vi "gyro-sweeper-module-V3.vi"(8 "fitter event pair":T4, 9 "async sweeper event pair":T4, 11 "this sweeper event pair":T4) -> ()   [LabVIEW 2018]
uses:
  filename-pattern.ctl
  show-win- control.ctl
  cursor winow.ctl
  server talk-to-back pair.ctl
  server talkback message type.ctl
  server talkto message type.ctl
  cursor window action.ctl
  pll internal user event action.ctl
  publisher action.ctl
  file -- read-write control.ctl
  KM_file -- read-write control.ctl
  filename-action.ctl
  <vilib>/Analysis/baseanly.llb/A x B.vi
  <vilib>/Analysis/baseanly.llb/Complex A x B.vi
  Q -- check range -- i -- real.vi
  line -- complex.vi
  Q -- check range -- i -- integer.vi
  Q - not nan -- real.vi
  Q - not nan -- integer.vi
  <vilib>/Analysis/Matrix/Numeric/Conversions/Array To Matrix.vi
  <vilib>/Analysis/Matrix/Numeric/Conversions/Array To Matrix - RA2.vi
  <vilib>/Analysis/baseanly.llb/Inverse Matrix.vi
  <vilib>/Analysis/baseanly.llb/Real Inverse Matrix.vi
panel:
  in  "view/hide fitter":bool
  in  "view/hide sweeper":bool=TRUE
  in  "sweeper panel":T1(tab)
  in  "sweep ON":bool
  in  "win":T2={"cen (Hz)"=32744.4, "win (Hz)"=134.34356253945762, "left (Hz)"=32677.228218730274, "right (Hz)"=32811.57178126973}
  out "Plot: circle sweep window":cluster{"Freq out (Hz)":dbl[], dbl[]}[](graph)
  in  "start/stop sweep: r":bool
  in  "subtract bgnd!":bool
  in  "fit!":bool=TRUE
  in  "cursor window":T3={"left"=32677.228218730274, "right "=32811.57178126973, "center"=32744.4, "window"=134.34356253945762, "cursors"=[0, 1, 2], "relative"=0, "absolute"=0, "fixed vertical offset"=0.0, "vertical offset"=0.0, "skew"=0.0, "default window frac"=0.1, "kind"=enum."symmetric", "skew.left"=0.5, "skew.right"=0.5, "Plot ref"=refnum, "wing order"=enum."forw"}
  in  "save data":enum32{"save/read"}(tab)
  in  "freqsweep name template":T5={"prefix"="RuCl3-rod", "group"="f"}
  in  "Save folder":path=path "/Users/Shared/Data"
  in  "freq sweep file name":string="f020_RuCl3-rod_042518.dat"
  in  "read from disk :l":bool
  in  "read file":path=path "/Users/arkady/Desktop/local_data/TaAs-quirk-Jan2018-losalamos/9w/f006_rucl3_012518.dat"
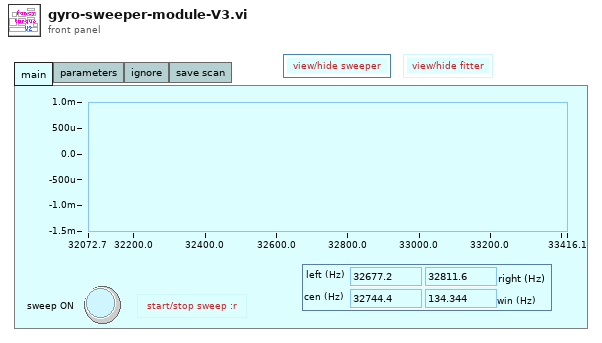
[diagram p1: front panel]
types:
  T1 = enum32{"main", "parameters", "ignore", "save scan"}
  T2 = typedef "show-win- control.ctl" = cluster{"cen (Hz)":dbl, "win (Hz)":dbl, "left (Hz)":dbl, "right (Hz)":dbl}
  T3 = typedef "cursor winow.ctl" = cluster{"left":dbl, "right ":dbl, "center":dbl, "window":dbl, "cursors":i32[], "relative":i32, "absolute":i32, "fixed vertical offset":dbl, "vertical offset":dbl, "skew":dbl, "default window frac":dbl, "kind":enum16{"symmetric", "skewed", "fancy"}, "skew.left":dbl, "skew.right":dbl, "Plot ref":refnum<vi>, "wing order":enum16{"forw", "back"}}
  T4 = typedef "server talk-to-back pair.ctl" = cluster{"talkback event":refnum<user-event>, "talkto event":refnum<user-event>}
  T5 = typedef "filename-pattern.ctl" = cluster{"prefix":string, "group":string}
  T6 = typedef "pll internal user event action.ctl" = enum16{"gear pll async", "start pll async", "stop pll async", "toggle pll async", "gear sweeper", "start sweeper", "stop sweeper", "toggle sweeper", "accept frequency", "reset lorentzian", "accept lorentzian", "update cursors", "pause pll", "unpause pll", "void", "exit", "gear server sweeper", "gear sweeper async", "gear fitter", "gear sourcer"}
  T7 = typedef "cursor window action.ctl" = enum16{"balance", "h. offset change", "cursor moves", "change center", "change window", "init", "check", "reset", "set y to middle", "idle", "-write all Y", "-write left.X", "-write center.X", "-write right.X", "-write all X", "-change center", "-change window", "-change skew", "-read cursor 2", "-read cursor 1", "-read cursor 0", "-read all cursors", "-reset", "-read plot scale", "-set y to middle", "-Q: center.Y is visible", "-Q: window is visible", "-parse center.Y", "-right left from center", "-left move", "-right move", "-set center.Y", "-empty", "-set cursors to default", "-check", "-write center.Y", "-copy cursor 1", "-copy cursor 0", "-copy cursor 2", "move right", "move left", "shrink", "broaden", "skew up", "skew down", "-write plot scale", "zoom X", "change cen&win", "zoom to all data", "color--red", "color--green", "color--yellow", "read", "zoom out", "zoom in", "slide right", "slide left", "set range aspect ratio to 1"}
  T8 = enum16{"stop", "start", "update pars", "update request", "new", "launch", "exit", "get", "reset", "pause", "unpause"}
  T9 = typedef "publisher action.ctl" = enum16{"set", "get", "init", "check"}
  T10 = typedef "file -- read-write control.ctl" = enum16{"read", "write all", "append one line"}
  T11 = typedef "filename-action.ctl" = enum16{"rewrite", "parse", "force pattern", "uniquenum"}
  T12 = typedef "KM_file -- read-write control.ctl" = enum16{"read", "write all", "append one line"}
  T13 = typedef "server talkto message type.ctl" = cluster{"message":enum16{"stop", "start", "update pars", "update request", "new", "launch", "exit", "get", "reset", "pause", "unpause"}}
  T14 = typedef "eventvkey.ctl" = enum16{"ASCII", "Enter", "Return", "Shift", "Ctrl", "Alt", "Cmd", "Opt", "Caps", "NumLock", "Clear", "Break", "Up", "Down", "Left", "Right", "Insert", "Delete", "Home", "End", "PageUp", "PageDown", "Escape", "Help", "Pause", "ScrollLock", "F1", "F2", "F3", "F4", "F5", "F6", "F7", "F8", "F9", "F10", "F11", "F12", "F13", "F14", "F15", "F16", "F17", "F18", "F19", "F20", "F21", "F22", "F23", "F24", "Play", "VolumeUp", "VolumeDown", "Mute", "Two Byte Char"}
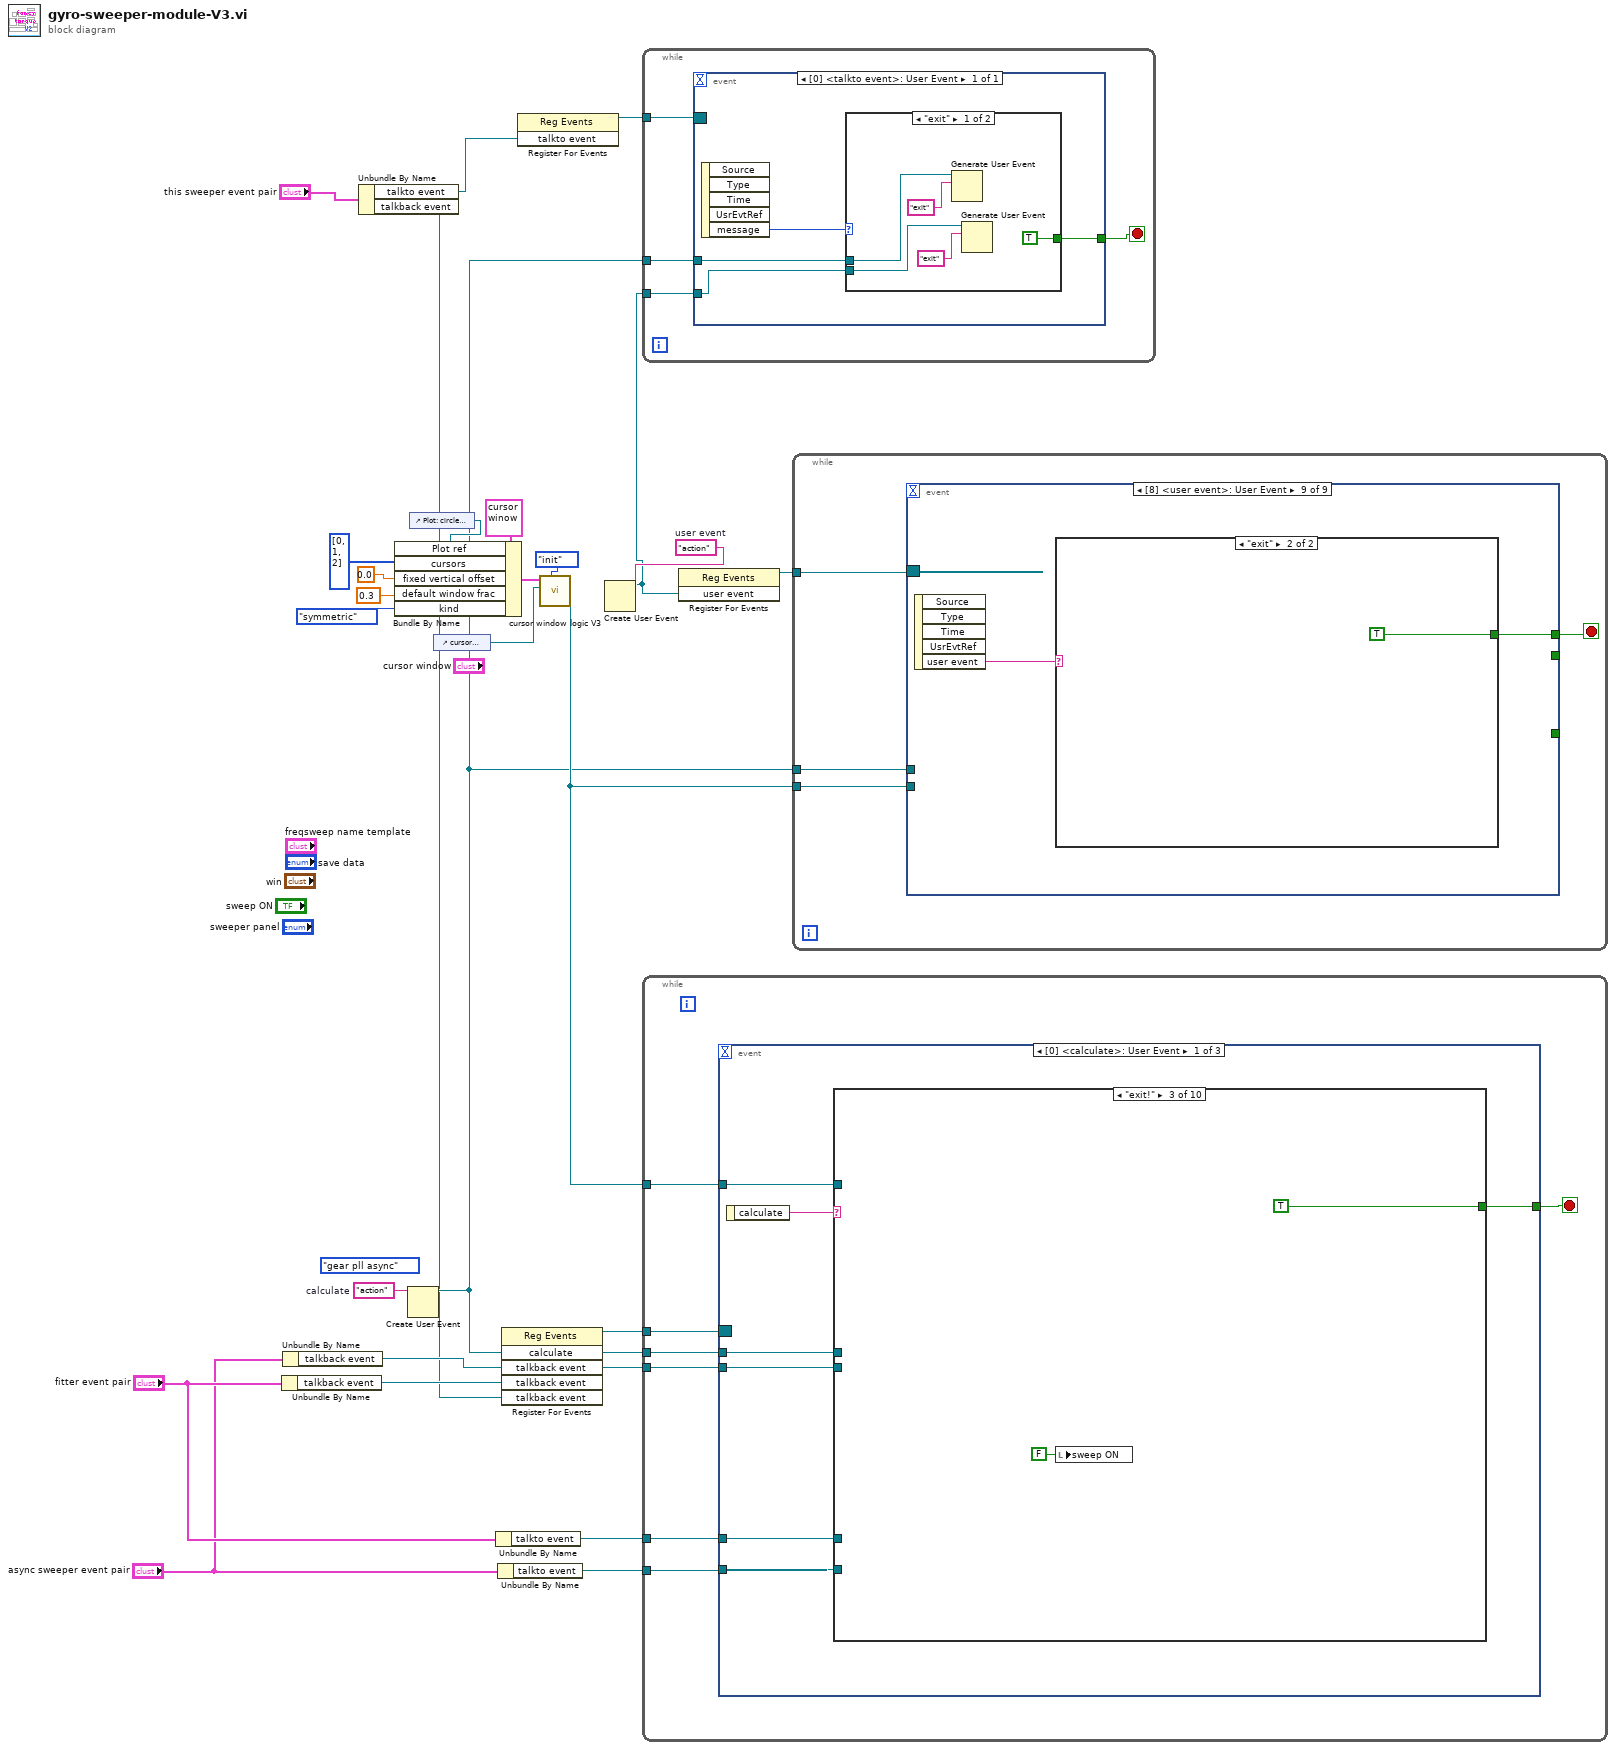
[diagram p0: block diagram]
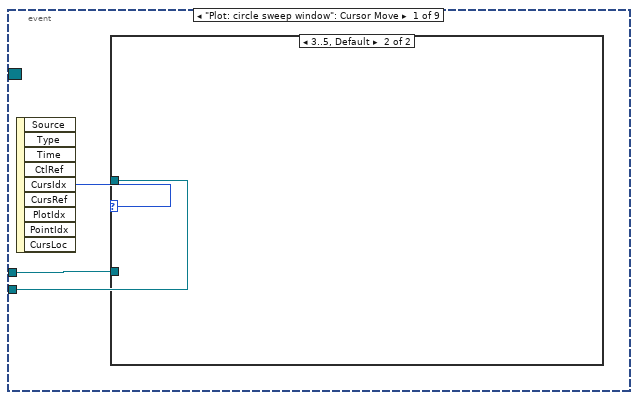
[diagram p3: hidden frame]
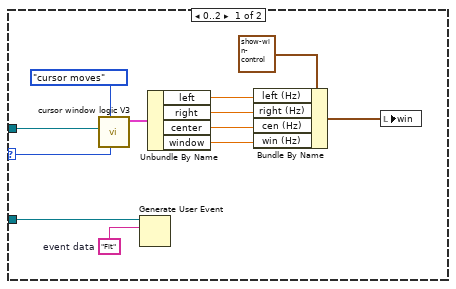
[diagram p4: hidden frame]
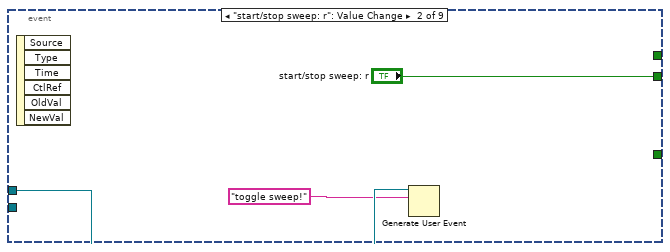
[diagram p5: hidden frame]
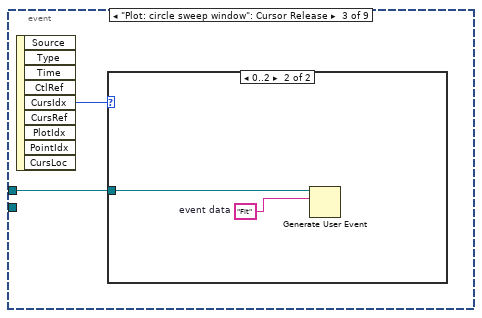
[diagram p6: hidden frame]
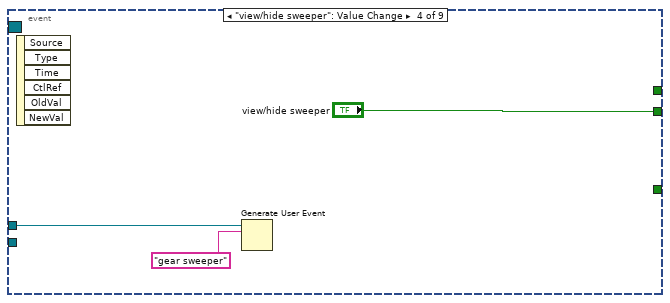
[diagram p8: hidden frame]
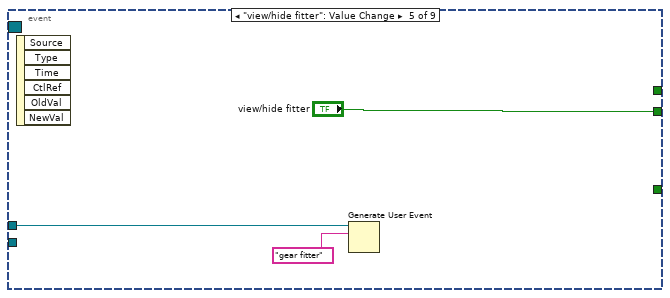
[diagram p9: hidden frame]
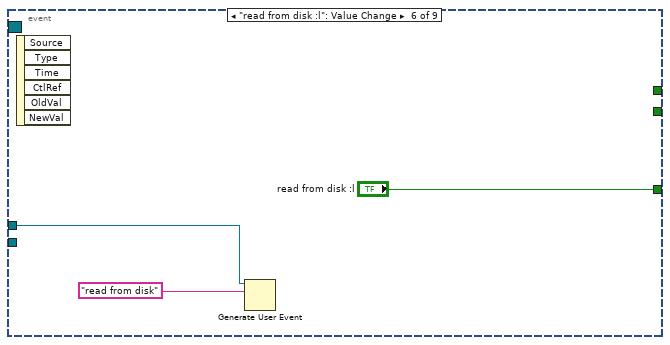
[diagram p10: hidden frame]
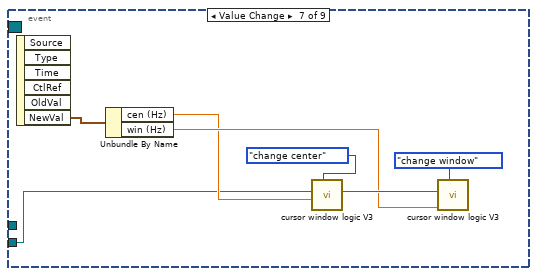
[diagram p11: hidden frame]
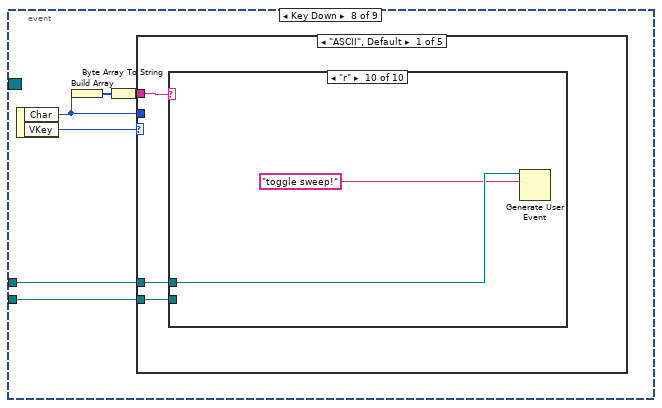
[diagram p12: hidden frame]
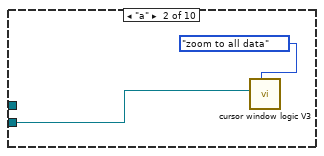
[diagram p14: hidden frame]
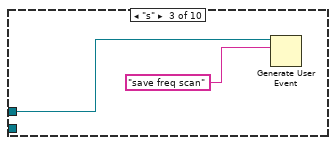
[diagram p15: hidden frame]
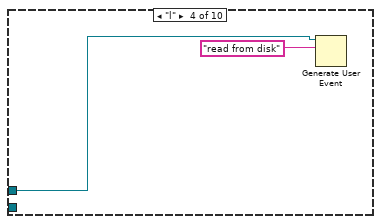
[diagram p16: hidden frame]
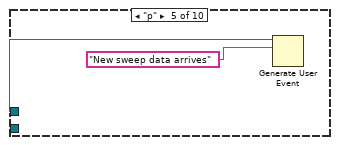
[diagram p17: hidden frame]
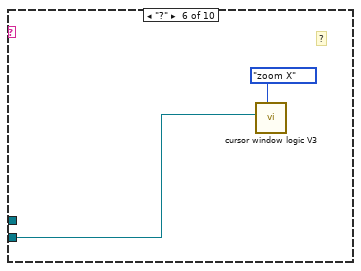
[diagram p18: hidden frame]
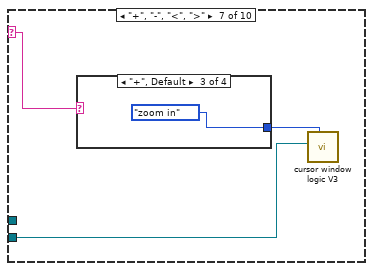
[diagram p19: hidden frame]
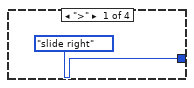
[diagram p20: hidden frame]
diagram:
  (unwired) pll_internal_user_event_action."gear pll async" ("pll event action")
  w23 = "action"  # user event
  w25 = "action"  # calculate
  n1 = Unbundle By Name("fitter event pair") -> ("talkback event"=w9:refnum<user-event>)
  n2 = Unbundle By Name("async sweeper event pair") -> ("talkback event"=w7:refnum<user-event>)
  n3 = Unbundle By Name("this sweeper event pair") -> ("talkto event"=w4:refnum<user-event>, "talkback event"=w1:refnum<user-event>)
  n4 = Create User Event(user event datatype=w25) -> (user event=w2:refnum<user-event>)  [unwired: 1 in, 1 out]
  n5 = control-ref of="Plot: circle sweep window"() -> (w14:refnum<vi>)
  n6 = Bundle By Name(cluster=T3 {"left"=0.0, "right "=0.0, "center"=0.0, "window"=0.0, "cursors"=[], "relative"=0, "absolute"=0, "fixed vertical offset"=0.0, "vertical offset"=0.0, "skew"=0.0, "default window frac"=0.0, "kind"=enum."symmetric", "skew.left"=0.0, "skew.right"=0.0, "Plot ref"=refnum, "wing order"=enum."forw"} ("cursor bracket: All, data window"), "Plot ref"=w14, "cursors"=i32[] [0, 1, 2], "fixed vertical offset"=0.0, "default window frac"=0.3 ("fixed vertical offset"), "kind"=enum16{"symmetric", "skewed", "fancy"}."symmetric") -> (w18:T3)
  n7 = control-ref of="cursor window"() -> (w13:refnum<vi>)
  n8 = Unbundle By Name("fitter event pair") -> ("talkto event"=w11:refnum<user-event>)
  n9 = Unbundle By Name("async sweeper event pair") -> ("talkto event"=w12:refnum<user-event>)
  n10 = register-events(w2, w7, w9, w1) -> (reference out=w26:refnum<event-registration>)  [unwired: 2 in, 1 out]
  n11 = register-events(w4) -> (reference out=w6:refnum<event-registration>)  [unwired: 2 in, 1 out]
  n12 = call "cursor window logic V3.vi"("cursor window action"=cursor_window_action."init", "cursor window in"=w13, "cursor window init"=w18) -> ("cursor window out"=w16:refnum<vi>)  [unwired: 7 in, 1 out]
  n13 = Create User Event(user event datatype=w23) -> (user event=w3:refnum<user-event>)  [unwired: 1 in, 1 out]
  n14 = while {
    tunnel: w6 -> [w30]
    tunnel: w2 -> [w28]
    tunnel: w3 -> [w27]
    stop <- w29 stop-if-true
    n15 = event shown="[0] <talkto event>: User Event" {
      selector: w30 -> [_]
      dyn-events: _ -> [_]
      timeout: _ -> [_]
      tunnel: [w33] -> w29
      tunnel: w28 -> [w32]
      tunnel: w27 -> [w31]
      event User Event {
        n16 = event-data() -> ("message"=w34:T8)  [unwired: 1 in, 4 out]
        n17 = case shown="\"exit\"" w34 {
          tunnel: [TRUE _] -> w33
          tunnel: w32 -> [w38 _]
          tunnel: w31 -> [w35 _]
          frame "exit" {
            n18 = Generate User Event(user event=w38, event data cluster="exit" ("event data")) -> ()  [unwired: 2 in, 2 out]
            n19 = Generate User Event(user event=w35, event data cluster="exit" ("event data")) -> ()  [unwired: 2 in, 2 out]
          }
          frame "start", Default {
          }
        }
      }
    }
  }
  n20 = while {
    tunnel: w26 -> [w46]
    tunnel: w2 -> [w45]
    tunnel: w16 -> [w44]
    tunnel: w12 -> [w43]
    tunnel: w7 -> [w42]
    tunnel: w11 -> [w41]
    stop <- w40 stop-if-true
    n21 = event shown="[0] <calculate>: User Event" {
      selector: w46 -> [_ _ _]
      dyn-events: _ -> [_ _ _]
      timeout: _ -> [_ _ _]
      tunnel: w45 -> [w52 w145 _]
      tunnel: w44 -> [w51 _ _]
      tunnel: w43 -> [w50 _ _]
      tunnel: w42 -> [w49 _ _]
      tunnel: w41 -> [w48 _ _]
      tunnel: [w47 _ _] -> w40
      event User Event {
        n22 = event-data() -> ("calculate"=w53:string)  [unwired: 1 in]
        n23 = case shown="\"exit!\"" w53 {
          tunnel: w52 -> [w62 w85 _ w90 _ _ _ _ _ _]
          tunnel: w51 -> [_ _ _ _ _ w122 _ _ _ _]
          tunnel: w50 -> [_ _ _ _ _ _ w135 w140 w144 _]
          tunnel: w49 -> [_ _ _ _ _ _ _ _ _ _]
          tunnel: w48 -> [_ _ _ _ _ w120 _ _ _ _]
          tunnel: [_ _ TRUE _ _ _ _ _ _ _] -> w47
          frame "New sweep data arrives" {
            n24 = call "MFLI -- publish -- freq scan.vi"("publisher action"=publisher_action."get") -> ("Voltage out (V)"=w59:cdb[], "Freq out (Hz)"=w61:dbl[])  [unwired: 9 in]
            n25 = Generate User Event(user event=w62, event data cluster="Fit" ("event data")) -> ()  [unwired: 2 in, 2 out]
            n26 = case shown="False" "subtract bgnd!" {
              tunnel: w61 -> [w74 w82]
              tunnel: [w68 w82] -> w60
              tunnel: w59 -> [w70 w81]
              tunnel: [w75 w81] -> w58
              frame True {
                w67 = 10 ("length")
                n27 = Delete From Array(array=w74, length=w67, index=0) -> (array with subset deleted=w73:dbl[])  [unwired: 1 out]
                n28 = Delete From Array(array=w70, length=w67, index=0) -> (array with subset deleted=w69:cdb[])  [unwired: 1 out]
                n29 = call "linear interp iiii- complex - z-omega.vi"("z"=w69, "omega"=w73) -> ("z out"=w76:cdb[], "omega out"=w68:dbl[], "intercept"=w78:cdb, "slope"=w79:cdb)  [unwired: 5 in, 5 out]
                n30 = Multiply(x=w68, y=w79) -> (x*y=w80:cdb[])
                n31 = Add(x=w80, y=w78) -> (x+y=w77:cdb[])
                n32 = Subtract(x=w76, y=w77) -> (x-y=w75:cdb[])
              }
              frame False {
              }
            }
            n33 = Complex To Re/Im(x + iy=w58) -> (x=w65:dbl[], y=w64:dbl[])
            n34 = Bundle("Freq out (Hz)"=w60, w65) -> (w66:cluster{"Freq out (Hz)":dbl[], dbl[]})  [unwired: 1 in]
            n35 = Bundle("Freq out (Hz)"=w60, w64) -> (w63:cluster{"Freq out (Hz)":dbl[], dbl[]})  [unwired: 1 in]
            n36 = Build Array(w66, w63) -> (→"Plot: circle sweep window":cluster{"Freq out (Hz)":dbl[], dbl[]}[])
          }
          frame "toggle sweep!" {
            n37 = local read "sweep ON"() -> (w84:bool)
            n38 = case shown="False" w84 {
              tunnel: ["start sweep!" ("event data") "stop sweep!" ("event data")] -> w83
              frame False {
              }
              frame True {
              }
            }
            n39 = Generate User Event(user event=w85, event data cluster=w83) -> ()  [unwired: 2 in, 2 out]
          }
          frame "exit!" {
            n40 = local write "sweep ON"(FALSE ("sweep ON")) -> ()
          }
          frame "read from disk" {
            n41 = call "file - read-write - list of lines.vi"("read/write control"=file_--_read-write_control."read", "file path"="read file") -> ("list of lines OUT"=w94:string[])  [unwired: 8 in, 1 out]
            n42 = for {
              tunnel: w94 -> [w104] mode=indexing
              tunnel: [w99] -> w95 mode=indexing
              tunnel: [w98] -> w96 mode=indexing
              w100 = 0.0
              n43 = Scan From String(format string="%f%f%f", input string=w104, default 1=w100, default 2=w100, default 3=w100) -> (output 1=w98:dbl, output 2=w102:dbl, output 3=w101:dbl)  [unwired: 2 in, 3 out]
              n44 = Re/Im To Complex(1:w101, 2:w102) -> (0:w99:cdb)
            }
            n45 = flat-sequence {
              tunnel: w90 -> [w108]
              tunnel: [w108] -> w97
              tunnel: w95 -> [w106]
              tunnel: w96 -> [w105]
              tunnel: w97 -> [w110]
              tunnel: "New sweep data arrives" ("event data") -> [w109]
              frame #0 {
                n46 = call "MFLI -- publish -- freq scan.vi"("publisher action"=publisher_action."set", "Voltage IN (V)"=w106, "Freq IN (Hz)"=w105) -> ()  [unwired: 7 in, 2 out]
              }
              frame #1 {
                n47 = Generate User Event(user event=w110, event data cluster=w109) -> ()  [unwired: 2 in, 2 out]
              }
            }
          }
          frame "save freq scan" {
            n48 = local read "freqsweep name template"() -> (w116:T5)
            n49 = call "MFLI -- publish -- freq scan.vi"("publisher action"=publisher_action."get") -> ("Voltage out (V)"=w112:cdb[], "Freq out (Hz)"=w113:dbl[])  [unwired: 9 in]
            n50 = call "filename-manage.vi"("filename pattern"=w116, "filename-action"=filename-action."uniquenum", "folder"="Save folder", "file name"="freq sweep file name") -> ("filename OUT"=w115:string)  [unwired: 7 in]
            n51 = call "KM_appendline -- freq sweep.vi"("freq"=w113, "Vout(V)"=w112, "Save frequency scan"="Save folder", "read/write control"=KM_file_--_read-write_control."append one line", "name or relative path"=w115) -> ()  [unwired: 15 in]
            n52 = local write "freq sweep file name"(w115) -> ()
          }
          frame "Fit" {
            n53 = case shown="True" "fit!" {
              tunnel: w122 -> [_ w124]
              tunnel: w120 -> [_ w123]
              frame False {
              }
              frame True {
                n54 = flat-sequence {
                  tunnel: w124 -> [w127]
                  tunnel: w123 -> [w129]
                  frame #0 {
                    n55 = call "cursor window logic V3.vi"("cursor window action"=cursor_window_action."read", "cursor window in"=w127) -> ("cursor window out"=w126:T3)  [unwired: 8 in, 1 out]
                    n56 = call "publish -- fitter window.vi"("publisher action"=publisher_action."set", "win IN"=w126) -> ()  [unwired: 9 in, 1 out]
                  }
                  frame #1 {
                    n57 = Generate User Event(user event=w129, event data cluster=T13 {"message"=enum."new"} ("event data")) -> ()  [unwired: 2 in, 2 out]
                  }
                }
              }
            }
          }
          frame "start sweep!" {
            n58 = local read "win"() -> (w132:T2)
            n59 = call "publish -- sweeper window.vi"("publisher action"=publisher_action."set", "win IN"=w132) -> ()  [unwired: 9 in, 1 out]
            n60 = local write "sweep ON"(TRUE ("sweep ON")) -> ()
            n61 = Generate User Event(user event=w135, event data cluster=T13 {"message"=enum."update request"} ("event data")) -> (user event out=w134:refnum<user-event>)  [unwired: 2 in, 1 out]
            n62 = Generate User Event(user event=w134, event data cluster=T13 {"message"=enum."start"} ("event data")) -> ()  [unwired: 2 in, 2 out]
          }
          frame "stop sweep!" {
            n63 = Generate User Event(user event=w140, event data cluster=T13 {"message"=enum."stop"} ("event data")) -> ()  [unwired: 2 in, 2 out]
            n64 = local write "sweep ON"(FALSE ("sweep ON")) -> ()
          }
          frame "update win" {
            n65 = local read "win"() -> (w141:T2)
            n66 = call "publish -- sweeper window.vi"("publisher action"=publisher_action."set", "win IN"=w141) -> ()  [unwired: 9 in, 1 out]
            n67 = Generate User Event(user event=w144, event data cluster=T13 {"message"=enum."update request"} ("event data")) -> ()  [unwired: 2 in, 2 out]
          }
          frame "Void", Default {
          }
        }
      }
      event User Event {
        n68 = event-data() -> ("message"=w146:enum16{"new", "void"})  [unwired: 1 in, 4 out]
        n69 = case shown="\"new\", Default" w146 {
          tunnel: w145 -> [w147]
          frame "new", Default {
            n70 = Generate User Event(user event=w147, event data cluster="New sweep data arrives" ("event data")) -> ()  [unwired: 2 in, 2 out]
          }
        }
      }
      event User Event {
        n71 = event-data() -> ()  [unwired: 1 in, 1 out]
      }
    }
  }
  n72 = register-events(w3) -> (reference out=w24:refnum<event-registration>)  [unwired: 2 in, 1 out]
  n73 = while {
    tunnel: w24 -> [w152]
    tunnel: w2 -> [w151]
    tunnel: w16 -> [w150]
    stop <- w149 stop-if-true
    n74 = event shown="[8] <user event>: User Event" {
      selector: w152 -> [_ _ _ _ _ _ _ _ _]
      dyn-events: _ -> [_ _ _ _ _ _ _ _ _]
      timeout: _ -> [_ _ _ _ _ _ _ _ _]
      tunnel: w151 -> [w153 w169 w172 w176 w178 w183 _ w195 _]
      tunnel: w150 -> [w155 _ _ _ _ _ w184 w191 _]
      tunnel: [_ "start/stop sweep: r" _ "view/hide sweeper" "view/hide fitter" _ _ _ _] -> _
      tunnel: [_ _ _ _ _ "read from disk :l" _ _ _] -> _
      tunnel: [_ _ _ _ _ _ _ _ w239] -> w149
      event "Plot: circle sweep window": Cursor Move {
        n75 = event-data() -> ("CursIdx"=w154:i32)  [unwired: 1 in, 8 out]
        n76 = case shown="3..5, Default" w154 {
          selector: w154 -> [w165 _]
          tunnel: w155 -> [w167 _]
          tunnel: w153 -> [w163 _]
          frame 0..2 {
            w162 = "Fit"  # event data
            n77 = call "cursor window logic V3.vi"("CursIdx"=w165, "cursor window action"=cursor_window_action."cursor moves", "cursor window in"=w167) -> ("cursor window out"=w164:T3)  [unwired: 7 in, 1 out]
            n78 = Generate User Event(user event=w163, event data cluster=w162) -> ()  [unwired: 2 in, 2 out]
            n79 = Unbundle By Name(w164) -> ("left"=w159:dbl, "right"=w158:dbl, "center"=w157:dbl, "window"=w156:dbl)
            n80 = Bundle By Name(cluster=T2 {"cen (Hz)"=-0.35260838541595674, "win (Hz)"=17.234446484426172, "left (Hz)"=-8.969831627629043, "right (Hz)"=8.26461485679713} ("win"), "left (Hz)"=w159, "right (Hz)"=w158, "cen (Hz)"=w157, "win (Hz)"=w156) -> (w160:T2)
            n81 = local write "win"(w160) -> ()
          }
          frame 3..5, Default {
          }
        }
      }
      event "start/stop sweep: r": Value Change {
        n82 = event-data() -> ()  [unwired: 1 in, 6 out]
        n83 = Generate User Event(user event=w169, event data cluster="toggle sweep!" ("event data")) -> ()  [unwired: 2 in, 2 out]
      }
      event "Plot: circle sweep window": Cursor Release {
        n84 = event-data() -> ("CursIdx"=w171:i32)  [unwired: 1 in, 8 out]
        n85 = case shown="0..2" w171 {
          tunnel: w172 -> [_ w173]
          frame 3, Default {
          }
          frame 0..2 {
            w174 = "Fit"  # event data
            n86 = Generate User Event(user event=w173, event data cluster=w174) -> ()  [unwired: 2 in, 2 out]
          }
        }
      }
      event "view/hide sweeper": Value Change {
        n87 = event-data() -> ()  [unwired: 1 in, 6 out]
        n88 = Generate User Event(user event=w176, event data cluster="gear sweeper" ("event data")) -> ()  [unwired: 2 in, 2 out]
      }
      event "view/hide fitter": Value Change {
        n89 = event-data() -> ()  [unwired: 1 in, 6 out]
        n90 = Generate User Event(user event=w178, event data cluster="gear fitter" ("event data")) -> ()  [unwired: 2 in, 2 out]
      }
      event "read from disk :l": Value Change {
        n91 = event-data() -> ()  [unwired: 1 in, 6 out]
        n92 = Generate User Event(user event=w183, event data cluster="read from disk" ("event data")) -> ()  [unwired: 2 in, 2 out]
      }
      event Value Change {
        n93 = event-data() -> ("NewVal"=w187:T2)  [unwired: 1 in, 5 out]
        n94 = Unbundle By Name(w187) -> ("cen (Hz)"=w185:dbl, "win (Hz)"=w186:dbl)
        n95 = call "cursor window logic V3.vi"("cursor window action"=cursor_window_action."change center", "center"=w185, "cursor window in"=w184) -> ("cursor window out"=w188:refnum<vi>)  [unwired: 7 in, 1 out]
        n96 = call "cursor window logic V3.vi"("cursor window action"=cursor_window_action."change window", "window"=w186, "cursor window in"=w188) -> ()  [unwired: 7 in, 2 out]
      }
      event Key Down {
        n97 = event-data() -> ("Char"=w193:i16, "VKey"=w196:T14)  [unwired: 1 in]
        n98 = Build Array(w193) -> (w194:i16[])
        n99 = Byte Array To String(unsigned byte array=w194) -> (string=w192:string)
        n100 = case shown="\"ASCII\", Default" w196 {
          selector: w196 -> [_ _ _ _ w234]
          tunnel: w193 -> [_ _ _ _ _]
          tunnel: w195 -> [w199 _ _ _ w233]
          tunnel: w192 -> [w198 _ _ _ _]
          tunnel: w191 -> [w197 _ _ _ w230]
          frame "ASCII", Default {
            n101 = case shown="\"r\"" w198 {
              selector: w198 -> [_ _ _ _ _ _ w211 _ _ _]
              tunnel: w199 -> [_ _ w202 w204 w206 _ _ _ _ w220]
              tunnel: w197 -> [_ w200 _ _ _ w208 w212 w217 _ _]
              frame "0", Default {
              }
              frame "a" {
                n102 = call "cursor window logic V3.vi"("cursor window action"=cursor_window_action."zoom to all data", "cursor window in"=w200) -> ()  [unwired: 8 in, 2 out]
              }
              frame "s" {
                n103 = Generate User Event(user event=w202, event data cluster="save freq scan" ("event data")) -> ()  [unwired: 2 in, 2 out]
              }
              frame "l" {
                n104 = Generate User Event(user event=w204, event data cluster="read from disk" ("event data")) -> ()  [unwired: 2 in, 2 out]
              }
              frame "p" {
                n105 = Generate User Event(user event=w206, event data cluster="New sweep data arrives" ("event data")) -> ()  [unwired: 2 in, 2 out]
              }
              frame "?" {
                # "?"
                n106 = call "cursor window logic V3.vi"("cursor window action"=cursor_window_action."zoom X", "cursor window in"=w208) -> ()  [unwired: 8 in, 2 out]
              }
              frame "+", "-", "<", ">" {
                n107 = case shown="\"+\", Default" w211 {
                  tunnel: [cursor_window_action."slide right" ("cursor window action") cursor_window_action."slide left" ("cursor window action") cursor_window_action."zoom in" ("cursor window action") cursor_window_action."zoom out" ("cursor window action")] -> w210
                  frame ">" {
                  }
                  frame "<" {
                  }
                  frame "+", Default {
                  }
                  frame "-" {
                  }
                }
                n108 = call "cursor window logic V3.vi"("cursor window action"=w210, "cursor window in"=w212) -> ()  [unwired: 8 in, 2 out]
              }
              frame "c" {
                n109 = call "cursor window logic V3.vi"("cursor window action"=cursor_window_action."check", "cursor window in"=w217) -> ()  [unwired: 8 in, 2 out]
              }
              frame "t" {
              }
              frame "r" {
                n110 = Generate User Event(user event=w220, event data cluster="toggle sweep!" ("event data")) -> ()  [unwired: 2 in, 2 out]
              }
            }
          }
          frame "Escape" {
          }
          frame "PageUp" {
          }
          frame "PageDown" {
          }
          frame "Up".."Right" {
            w221 = "update win"  # event data
            w223 = "Fit"  # event data
            n111 = case shown="\"Left\"" w234 {
              tunnel: [cursor_window_action."move right" ("cursor window action") cursor_window_action."move left" ("cursor window action") cursor_window_action."broaden" ("cursor window action") cursor_window_action."shrink" ("cursor window action")] -> w232
              frame "Right", Default {
              }
              frame "Left" {
              }
              frame "Up" {
              }
              frame "Down" {
              }
            }
            n112 = call "cursor window logic V3.vi"("cursor window action"=w232, "cursor window in"=w230) -> ("cursor window out"=w231:T3)  [unwired: 8 in, 1 out]
            n113 = Unbundle By Name(w231) -> ("left"=w227:dbl, "right"=w226:dbl, "center"=w225:dbl, "window"=w224:dbl)
            n114 = Generate User Event(user event=w233, event data cluster=w223) -> (user event out=w222:refnum<user-event>)  [unwired: 2 in, 1 out]
            n115 = Bundle By Name(cluster=T2 {"cen (Hz)"=-0.35260838541595674, "win (Hz)"=17.234446484426172, "left (Hz)"=-8.969831627629043, "right (Hz)"=8.26461485679713} ("win"), "left (Hz)"=w227, "right (Hz)"=w226, "cen (Hz)"=w225, "win (Hz)"=w224) -> (w229:T2)
            n116 = Generate User Event(user event=w222, event data cluster=w221) -> ()  [unwired: 2 in, 2 out]
            n117 = local write "win"(w229) -> ()
          }
        }
      }
      event User Event {
        n118 = event-data() -> ("user event"=w240:string)  [unwired: 1 in, 4 out]
        n119 = case shown="\"exit\"" w240 {
          tunnel: [_ TRUE] -> w239
          frame "False", Default {
          }
          frame "exit" {
          }
        }
      }
    }
  }
